vi "Image UDP Broadcast Main Page.vi"(8 "error in (no error)":errorcluster, 11 "Node Ptr":T4 format="%.0x") -> (0 "error out":errorcluster)   [LabVIEW 2012, in "Image UDP Broadcast Custom Device.lvlib"]
uses:
  Shared/Image UDP Broadcast Custom Device.lvlib
  <vilib>/NI Veristand/Custom Device API/Custom Device Item Ref.ctl
  Ctls/Acquisition States.ctl
  Ctls/Acquisition Data.ctl
  <vilib>/userdefined/High Color/IMAQdx.ctl
  <vilib>/vision/Image Controls.llb/IMAQ Image.ctl
  Shared/Image UDP Broadcast Global Variable.vi
  <vilib>/NI Veristand/Custom Device API/Custom Device API.lvlib
  <vilib>/vision/driver/NI_Vision_Acquisition_Software.lvlib
panel:
  out "Valid Bytes per Packet":bool
  in  "Remote IP Address":string
  out "Camera State":T1
  in  "Image Type":T2 items=["Grayscale (U8)", "Grayscale (I16)", "Grayscale (SGL)", "Complex (CSG)", "RGB (U32)", "HSL (U32)", "RGB (U64)", "Grayscale (U16)"]
  in  "Quality":i32 min=0 max=1000 step=5
  out "% Bytes per Packet":dbl
  in  "UDP Port":u16
  in  "Discover IMAQdx":bool
  in  "NI-IMAQdx Devices":i32(listbox)
  in  "Camera Interface":string="cam0"
  in  "Grab":bool
  out "Image":T3(plugin-control)
  in  "Header":cluster{"Section Name":string}={"Section Name"="Custom Device Item Settings"}
  in  "Name":string
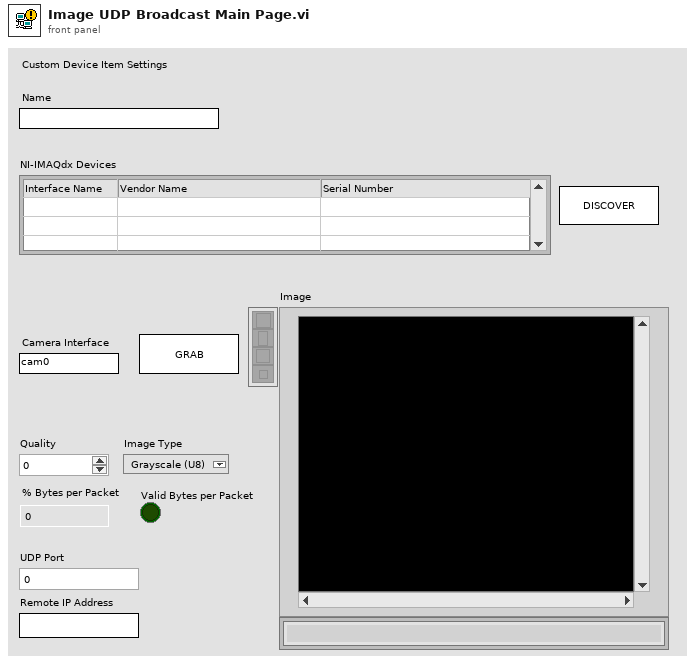
[diagram p1: front panel]
types:
  T1 = typedef "Image UDP Broadcast Custom Device.lvlib/Acquisition States.ctl" = enum8{"Idle", "Init & Config", "Acq", "Stop"}
  T2 = typedef "Image Type" = u32
  T3 = typedef "IMAQ Image.ctl" = refnum<image>
  T4 = typedef "Custom Device API.lvlib/Custom Device Item Ref.ctl" = u64
  T5 = typedef "Image UDP Broadcast Custom Device.lvlib/Acquisition Data.ctl" = cluster{"State":T1, "IMAQdx Session":T6, "Image":T3, "% Bytes per Packet":dbl}
  T6 = typedef "IMAQdx.ctl" = refnum<k21>
  T7 = typedef "Custom Device API.lvlib/Custom Device Item Info.ctl" = cluster{"Name":string, "Is Channel":bool, "GUID":string, "Is Waveform":bool}
  T8 = typedef "Custom Device API.lvlib/Custom Device Commands.ctl" = enum16{"Default", "Item renamed", "Shutdown", "Dynamic button pressed"}
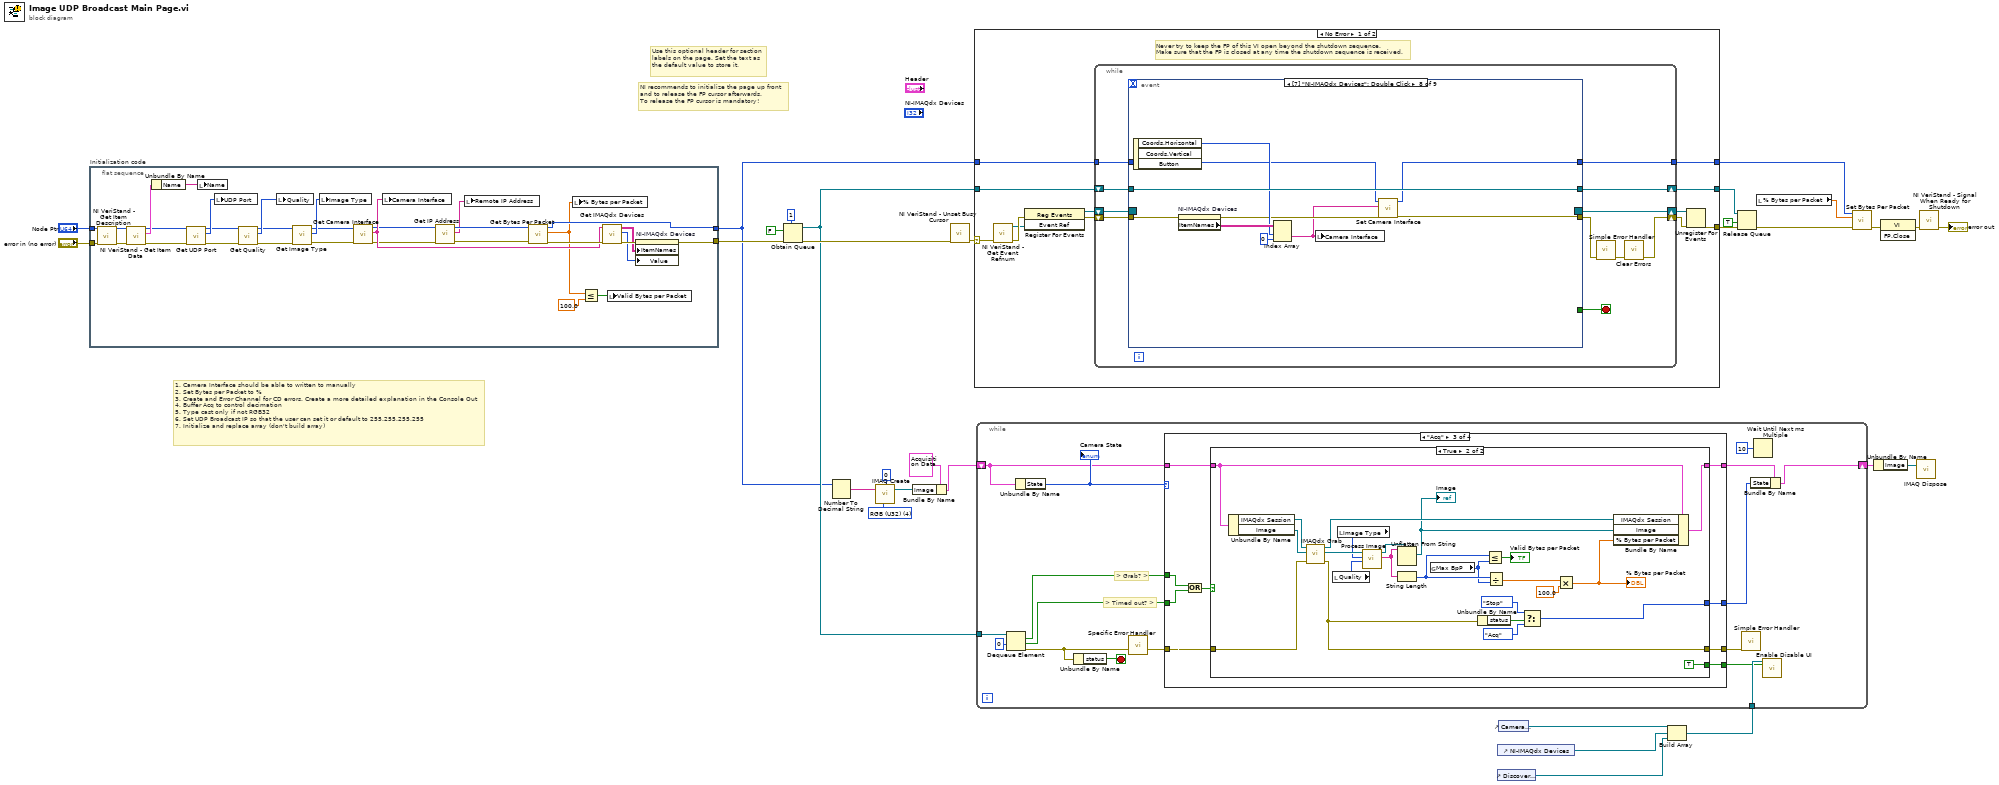
[diagram p0: block diagram]
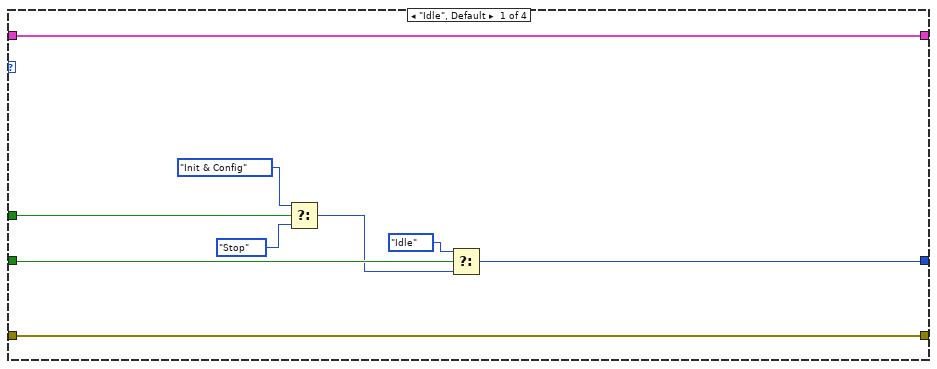
[diagram p2: hidden frame]
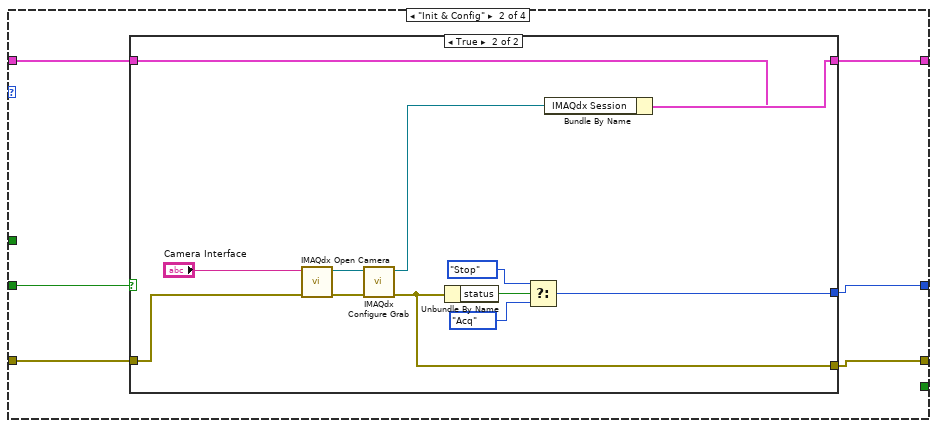
[diagram p3: hidden frame]
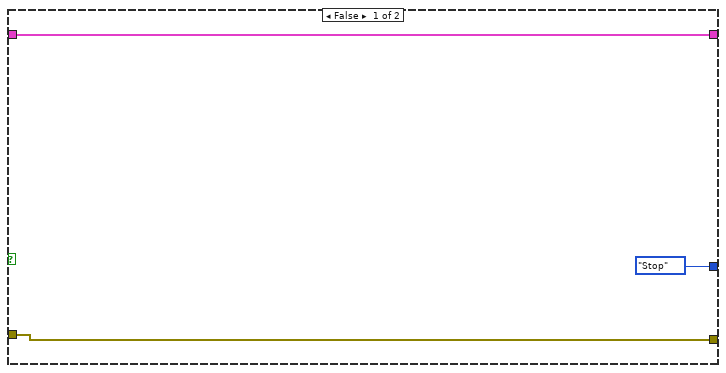
[diagram p4: hidden frame]
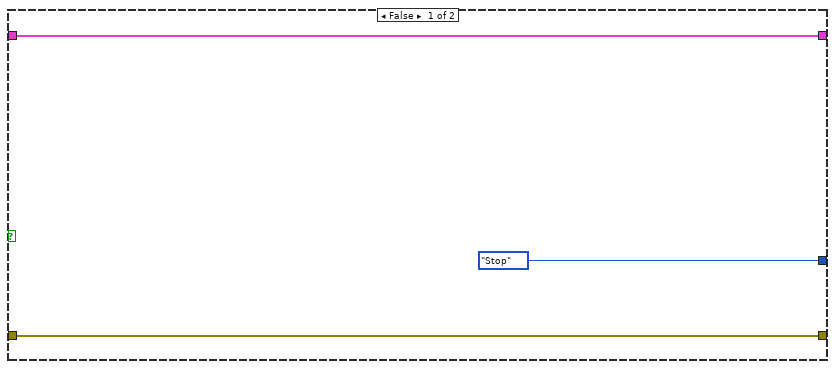
[diagram p5: hidden frame]
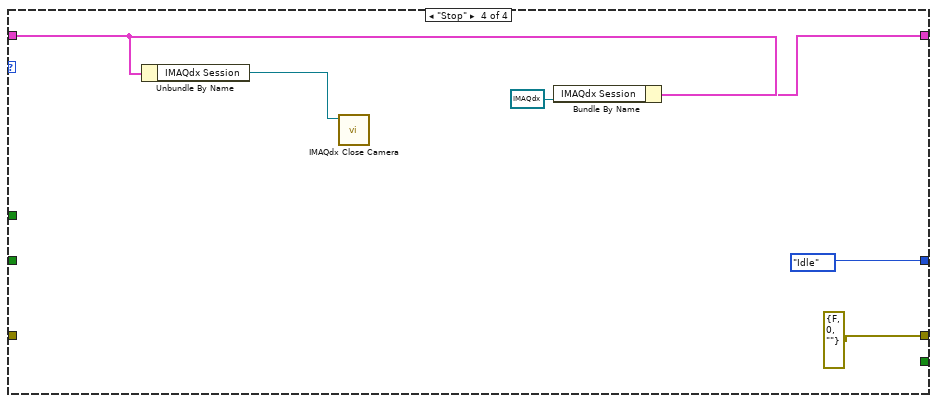
[diagram p6: hidden frame]
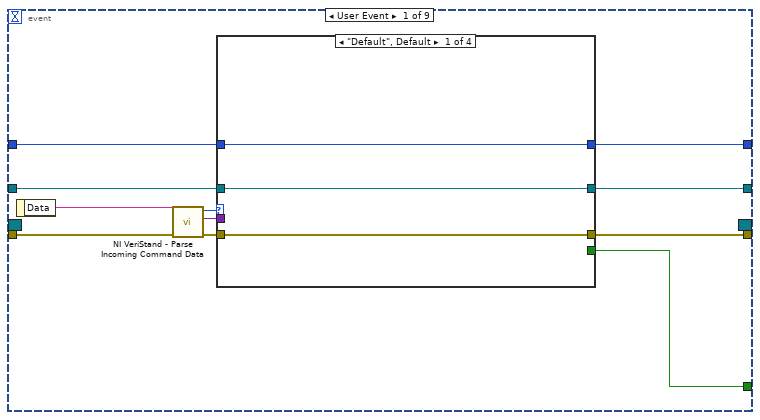
[diagram p7: hidden frame]
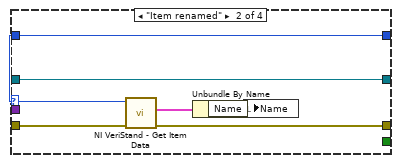
[diagram p8: hidden frame]
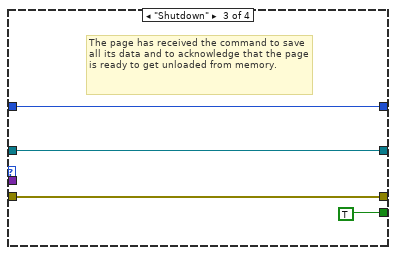
[diagram p9: hidden frame]
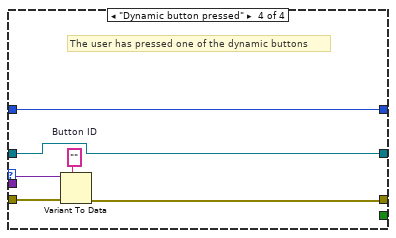
[diagram p10: hidden frame]
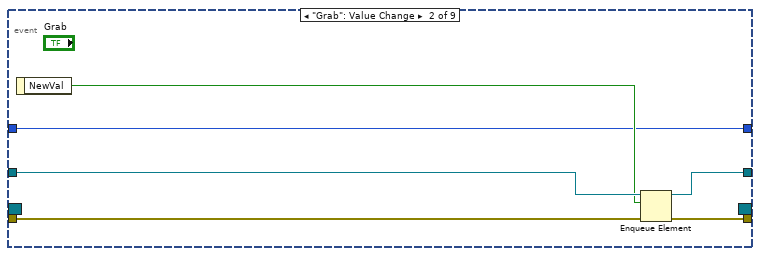
[diagram p11: hidden frame]
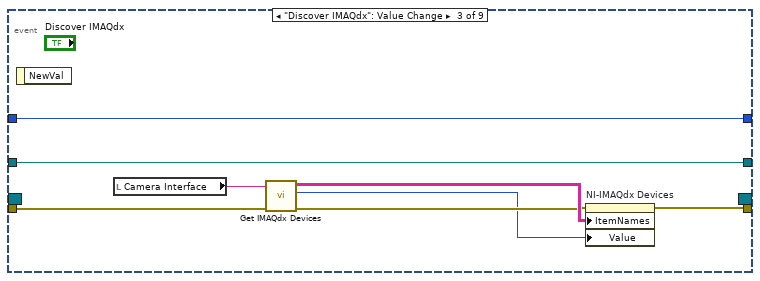
[diagram p12: hidden frame]
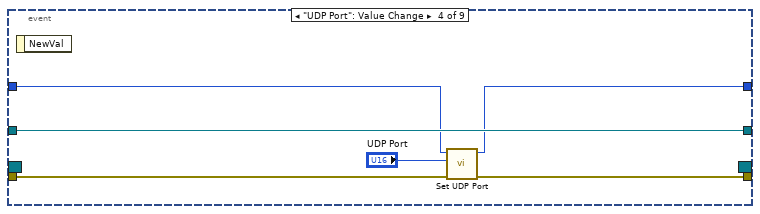
[diagram p13: hidden frame]
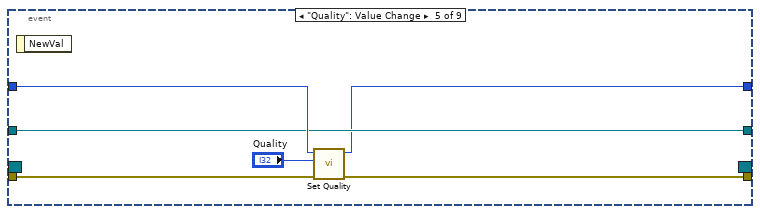
[diagram p14: hidden frame]
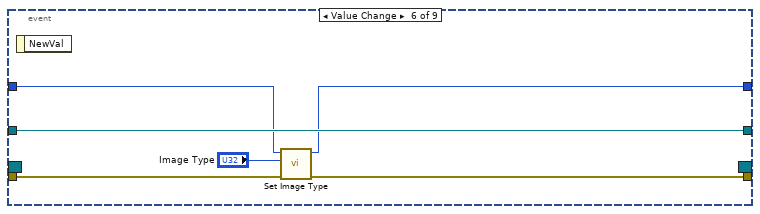
[diagram p15: hidden frame]
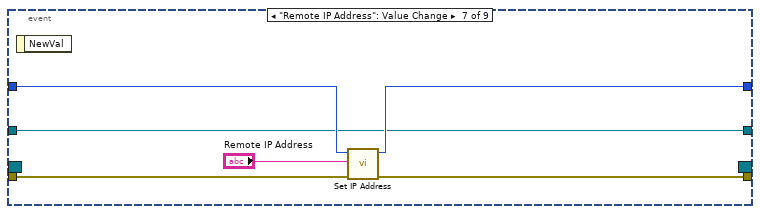
[diagram p16: hidden frame]
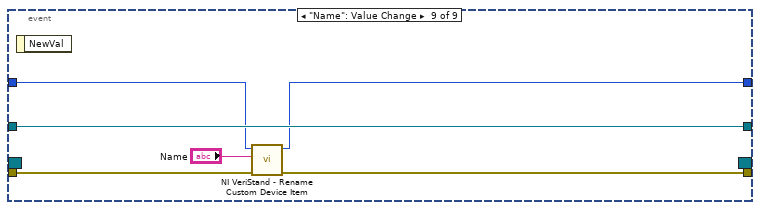
[diagram p17: hidden frame]
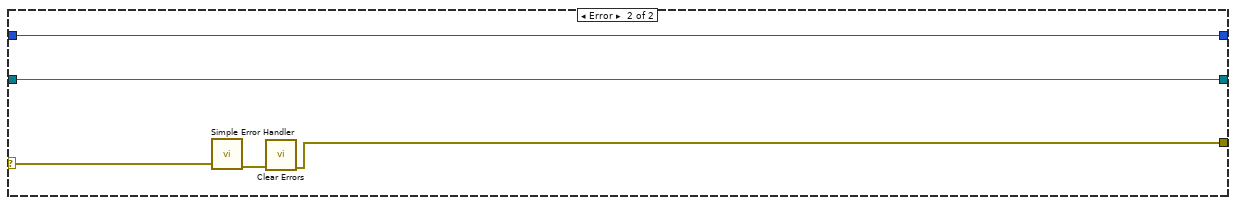
[diagram p18: hidden frame]
diagram:
  w10 = T2 4 items=["Grayscale (U8)", "Grayscale (I16)", "Grayscale (SGL)", "Complex (CSG)", "RGB (U32)", "HSL (U32)", "RGB (U64)", "Grayscale (U16)"] ("Image Type")
  # "1. Camera Interface should be able to written to manually\n2. Set Bytes per Packet to % \n3. Create and Error Channel for CD errors. Create a more detailed explanation in the Console Out\n4. Buffer Acq to control decimation\n5. Type cast only if not RGB32\n6. Set UDP Broadcast IP so that the user can set it or default to 255.255.255.255\n7. Initialize and replace array (don't build array)"
  # "Use this optional header for section labels on the page. Set the text as the default value to store it."
  # "NI recommends to initialize the page up front\nand to release the FP cursor afterwards.\nTo release the FP cursor is mandatory!"
  n1 = flat-sequence "Initialization code" {
    tunnel: "error in (no error)" -> [w60]
    tunnel: "Node Ptr" -> [w59]
    tunnel: [w33] -> w23
    tunnel: [w44] -> w16
    frame #0 {
      n2 = call <vilib>:"NI VeriStand - Get Item Description.vi"("error in (no error)"=w60, "Item Ref in"=w59) -> ("error out"=w58:errorcluster, "Item Ref out"=w61:T4)  [unwired: 8 out]
      n3 = call <vilib>:"NI VeriStand - Get Item Data.vi"("error in (no error)"=w58, "Item Ref in"=w61) -> ("error out"=w54:errorcluster, "Item Info"=w57:T7, "Item Ref out"=w55:T4)  [unwired: 7 out]
      n4 = Unbundle By Name(w57) -> ("Name"=w56:string)
      n5 = call "Get UDP Port.vi"("error in (no error)"=w54, "Dev Ref in"=w55) -> ("error out"=w52:errorcluster, "Value"=w53:u16, "Dev Ref out"=w51:T4)  [unwired: 7 in]
      n6 = local write "Name"(w56) -> ()
      n7 = local write "UDP Port"(w53) -> ()
      n8 = call "Get Quality.vi"("error in (no error)"=w52, "Dev Ref in"=w51) -> ("error out"=w49:errorcluster, "Value"=w50:i32, "Dev Ref out"=w48:T4)  [unwired: 7 in]
      n9 = local write "Quality"(w50) -> ()
      n10 = call "Get Image Type.vi"("error in (no error)"=w49, "Dev Ref in"=w48) -> ("error out"=w45:errorcluster, "Value"=w47:T2, "Dev Ref out"=w46:T4)  [unwired: 7 in]
      n11 = local write "Image Type"(w47) -> ()
      n12 = call "Get Camera Interface.vi"("error in (no error)"=w45, "Dev Ref in"=w46) -> ("error out"=w38:errorcluster, "Value"=w39:string, "Dev Ref out"=w37:T4)  [unwired: 7 in]
      n13 = local write "Camera Interface"(w39) -> ()
      n14 = call "Get IP Address.vi"("error in (no error)"=w38, "Dev Ref in"=w37) -> ("error out"=w35:errorcluster, "Value"=w34:string, "Dev Ref out"=w36:T4)  [unwired: 7 in]
      n15 = local write "Remote IP Address"(w34) -> ()
      n16 = call "Get Bytes Per Packet.vi"("error in (no error)"=w35, "Dev Ref in"=w36) -> ("error out"=w42:errorcluster, "Value"=w32:dbl, "Dev Ref out"=w44:T4)  [unwired: 7 in]
      n17 = local write "% Bytes per Packet"(w32) -> ()
      n18 = Less Or Equal?(x=w32, y=100.0) -> (x <= y?=w30:bool)
      n19 = call "Get IMAQdx Devices.vi"("error in (no error)"=w42, "Chosen Interface"=w39) -> ("error out"=w43:errorcluster, "Row of Chosen Interface"=w40:i32, "IMAQdx Devices"=w41:string[][])  [unwired: 6 in, 1 out]
      n20 = local write "Valid Bytes per Packet"(w30) -> ()
      n21 = property on="NI-IMAQdx Devices" class="MCListbox (strict)"(error in=w43, "ItemNames"=w41, "Value"=w40) -> (error out=w33:errorcluster)  [unwired: 1 in, 1 out]
    }
  }
  n22 = Obtain Queue(max queue size (-1, unlimited)=1, element data type=FALSE ("Grab"), error in (no error)=w23) -> (queue out=w17:refnum<queue>, error out=w18:errorcluster)  [unwired: 2 in, 1 out]
  n23 = Number To Decimal String(number=w16) -> (decimal integer string=w8:string)  [unwired: 1 in]
  n24 = call "IMAQ Create"("Border Size"=0, "Image Name"=w8, "Image Type"=w10) -> ("New Image"=w7:T3)  [unwired: 2 in, 1 out]
  n25 = Bundle By Name(cluster=T5 {"State"=enum."Idle", "IMAQdx Session"="", "Image"=refnum, "% Bytes per Packet"=0.0}, "Image"=w7) -> (w11:T5)
  n26 = call <vilib>:"NI VeriStand - Unset Busy Cursor.vi"("error in (no error)"=w18) -> ("error out"=w26:errorcluster)  [unwired: 10 out]
  n27 = case shown="No Error" w26 {
    selector: w26 -> [w65 w173]
    tunnel: [w70 w171] -> w21
    tunnel: w16 -> [w66 w169]
    tunnel: w17 -> [w64 w170]
    tunnel: [w63 w170] -> w20
    tunnel: [w62 w169] -> w4
    frame No Error {
      # "Never try to keep the FP of this VI open beyond the shutdown sequence.\nMake sure that the FP is closed at any time the shutdown sequence is received."
      n28 = call <vilib>:"NI VeriStand - Get Event Refnum.vi"("error in (no error)"=w65) -> ("error out"=w73:errorcluster, "Event Ref"=w69:refnum<user-event>)  [unwired: 9 out]
      n29 = register-events(error in=w73, w69) -> (reference out=w67:refnum<event-registration>, error out=w68:errorcluster)  [unwired: 1 in]
      n30 = while {
        tunnel: w66 -> [w80]
        shift-right: [w77] -> w71
        shift-left: w68 -> [w83]
        shift-right: [w84] -> w72
        shift-left: w67 -> [w82]
        shift-right: [w75] -> w63
        shift-left: w64 -> [w76]
        tunnel: [w74] -> w62
        stop <- w81 stop-if-true
        n31 = event shown="[7] \"NI-IMAQdx Devices\": Double Click" {
          selector: w82 -> [_ _ _ _ _ _ _ _ _]
          dyn-events: [_ _ _ _ _ _ _ _ _] -> w84
          timeout: _ -> [_ _ _ _ _ _ _ _ _]
          tunnel: w83 -> [w95 w115 w127 w133 w140 w146 w152 w162 w168]
          tunnel: [w91 _ _ _ _ _ _ _ _] -> w81
          tunnel: [w90 w118 w124 w132 w139 w145 w149 w156 w167] -> w79
          tunnel: w80 -> [w89 w116 w123 w131 w138 w143 w151 w154 w164]
          tunnel: w76 -> [w86 w120 w128 w134 w136 w144 w148 w159 w165]
          tunnel: [w85 w119 w128 w134 w136 w144 w148 w159 w165] -> w75
          tunnel: [w87 w116 w123 w129 w135 w141 w150 w153 w163] -> w74
          event User Event {
            n32 = event-data() -> ("Data"=w94:string)  [unwired: 1 out]
            n33 = call <vilib>:"NI VeriStand - Parse Incoming Command Data.vi"("error in (no error)"=w95, "Incoming data"=w94) -> ("error out"=w93:errorcluster, "Outgoing data"=w88:variant, "Action"=w92:T8)  [unwired: 7 out]
            n34 = case shown="\"Default\", Default" w92 {
              tunnel: w93 -> [w98 w104 w105 w114]
              tunnel: [_ _ TRUE _] -> w91
              tunnel: [w98 w102 w105 w111] -> w90
              tunnel: w89 -> [w97 w100 w107 w110]
              tunnel: w88 -> [_ _ _ w113]
              tunnel: [w97 w100 w107 w110] -> w87
              tunnel: w86 -> [w96 w99 w106 w109]
              tunnel: [w96 w99 w106 w109] -> w85
              frame "Default", Default {
              }
              frame "Item renamed" {
                n35 = call <vilib>:"NI VeriStand - Get Item Data.vi"("error in (no error)"=w104, "Item Ref in"=w100) -> ("error out"=w102:errorcluster, "Item Info"=w103:T7)  [unwired: 8 out]
                n36 = Unbundle By Name(w103) -> ("Name"=w101:string)
                n37 = local write "Name"(w101) -> ()
              }
              frame "Shutdown" {
                # "The page has received the command to save all its data and to acknowledge that the page is ready to get unloaded from memory."
              }
              frame "Dynamic button pressed" {
                w112 = ""  # Button ID
                # "The user has pressed one of the dynamic buttons"
                n38 = Variant To Data(error in=w114, type=w112, Variant=w113) -> (error out=w111:errorcluster)  [unwired: 1 out]
              }
            }
          }
          event "Grab": Value Change {
            n39 = event-data() -> ("NewVal"=w117:bool)  [unwired: 1 out]
            n40 = Enqueue Element(queue=w120, element=w117, error in (no error)=w115) -> (queue out=w119:refnum<queue>, error out=w118:errorcluster)  [unwired: 1 in, 1 out]
          }
          event "Discover IMAQdx": Value Change {
            n41 = event-data() -> ()  [unwired: 2 out]
            n42 = local read "Camera Interface"() -> (w121:string)
            n43 = call "Get IMAQdx Devices.vi"("error in (no error)"=w127, "Chosen Interface"=w121) -> ("error out"=w125:errorcluster, "Row of Chosen Interface"=w122:i32, "IMAQdx Devices"=w126:string[][])  [unwired: 6 in, 1 out]
            n44 = property on="NI-IMAQdx Devices" class="MCListbox (strict)"(error in=w125, "ItemNames"=w126, "Value"=w122) -> (error out=w124:errorcluster)  [unwired: 1 in, 1 out]
          }
          event "UDP Port": Value Change {
            n45 = event-data() -> ()  [unwired: 2 out]
            n46 = call "Set UDP Port.vi"("error in (no error)"=w133, "Value"="UDP Port", "Dev Ref in"=w131) -> ("error out"=w132:errorcluster, "Dev Ref out"=w129:T4)  [unwired: 7 in]
          }
          event "Quality": Value Change {
            n47 = event-data() -> ()  [unwired: 2 out]
            n48 = call "Set Quality.vi"("error in (no error)"=w140, "Value"="Quality", "Dev Ref in"=w138) -> ("error out"=w139:errorcluster, "Dev Ref out"=w135:T4)  [unwired: 7 in]
          }
          event Value Change {
            n49 = event-data() -> ()  [unwired: 2 out]
            n50 = call "Set Image Type.vi"("error in (no error)"=w146, "Value"="Image Type", "Dev Ref in"=w143) -> ("error out"=w145:errorcluster, "Dev Ref out"=w141:T4)  [unwired: 7 in]
          }
          event "Remote IP Address": Value Change {
            n51 = event-data() -> ()  [unwired: 2 out]
            n52 = call "Set IP Address.vi"("error in (no error)"=w152, "Value"="Remote IP Address", "Dev Ref in"=w151) -> ("error out"=w149:errorcluster, "Dev Ref out"=w150:T4)  [unwired: 7 in]
          }
          event "NI-IMAQdx Devices": Double Click {
            n53 = event-data() -> ("Coords.Horizontal"=w158:i32)  [unwired: 3 out]
            n54 = property on="NI-IMAQdx Devices" class="MCListbox (strict)"(error in=w162) -> (error out=w157:errorcluster, "ItemNames"=w161:string[][])  [unwired: 1 in, 1 out]
            n55 = Index Array(array=w161, index (row)=w158, index (col)=0 ("disabled index (col)")) -> (element=w155:string)
            n56 = local write "Camera Interface"(w155) -> ()
            n57 = call "Set Camera Interface.vi"("error in (no error)"=w157, "Value"=w155, "Dev Ref in"=w154) -> ("error out"=w156:errorcluster, "Dev Ref out"=w153:T4)  [unwired: 7 in]
          }
          event "Name": Value Change {
            n58 = event-data() -> ()  [unwired: 2 out]
            n59 = call <vilib>:"NI VeriStand - Rename Custom Device Item.vi"("error in (no error)"=w168, "New Name"="Name", "Item Ref in"=w164) -> ("error out"=w167:errorcluster, "Item Ref out"=w163:T4)  [unwired: 1 in, 6 out]
          }
        }
        n60 = call <vilib>:"Simple Error Handler.vi"("error in (no error)"=w79) -> ("error out"=w78:errorcluster)  [unwired: 1 in, 7 out]
        n61 = call <vilib>:"Clear Errors.vi"("error in (no error)"=w78) -> ("error out"=w77:errorcluster)  [unwired: 6 out]
      }
      n62 = Unregister For Events(event registration refnum=w72, error in=w71) -> (error out=w70:errorcluster)
    }
    frame Error {
      n63 = call <vilib>:"Simple Error Handler.vi"("error in (no error)"=w173) -> ("error out"=w172:errorcluster)  [unwired: 1 in, 7 out]
      n64 = call <vilib>:"Clear Errors.vi"("error in (no error)"=w172) -> ("error out"=w171:errorcluster)  [unwired: 6 out]
    }
  }
  n65 = control-ref of="NI-IMAQdx Devices"() -> (w14:refnum<vi>)
  n66 = control-ref of="Discover IMAQdx"() -> (w13:refnum<vi>)
  n67 = control-ref of="Camera Interface"() -> (w15:refnum<vi>)
  n68 = Build Array(w15, w14, w13) -> (w2:refnum<vi>[])
  n69 = while {
    tunnel: w17 -> [w188]
    shift-right: [w181] -> w6
    shift-left: w11 -> [w178]
    tunnel: w2 -> [w175]
    stop <- w184 stop-if-true
    # "> Grab? >"
    # "> Timed out? >"
    n70 = Dequeue Element(queue=w188, timeout in ms (-1)=0) -> (element=w185:bool, timed out?=w186:bool, error out=w177:errorcluster)  [unwired: 1 in, 1 out]
    n71 = Unbundle By Name(w178) -> ("State"=w179:T1)
    "Camera State" <- w179
    n72 = Unbundle By Name(w177) -> ("status"=w184:bool)
    n73 = call "Specific Error Handler"("Error to Check"=w177) -> ("error out"=w176:errorcluster)  [unwired: 11 in, 3 out]
    n74 = case shown="\"Acq\"" w179 {
      tunnel: w186 -> [w198 w203 w227 _]
      tunnel: w176 -> [w191 w204 w228 _]
      tunnel: w185 -> [w196 _ w225 _]
      tunnel: w178 -> [w190 w202 w223 w259]
      tunnel: [w190 w201 w222 w258] -> w183
      tunnel: [w192 w200 w224 Acquisition_States."Idle"] -> w182
      tunnel: [w191 w199 w221 errorcluster {"status"=FALSE, "code"=0, "source"=""} ("error out")] -> w180
      tunnel: [_ _ w220 _] -> w174
      frame "Idle", Default {
        n75 = Select(t=Acquisition_States."Init & Config", s=w196, f=Acquisition_States."Stop") -> (s? t:f=w193:T1)
        n76 = Select(t=Acquisition_States."Idle", s=w198, f=w193) -> (s? t:f=w192:T1)
      }
      frame "Init & Config" {
        n77 = case shown="True" w203 {
          tunnel: w204 -> [w206 w217]
          tunnel: [Acquisition_States."Stop" w216] -> w200
          tunnel: w202 -> [w205 w208]
          tunnel: [w205 w215] -> w201
          tunnel: [w206 w212] -> w199
          frame False {
          }
          frame True {
            n78 = call <vilib>:"IMAQdx Open Camera.vi"("error in"=w217, "Session In"="Camera Interface") -> ("error out"=w214:errorcluster, "Session Out"=w213:T6)  [unwired: 8 in]
            n79 = call <vilib>:"IMAQdx Configure Grab.vi"("error in"=w214, "Session In"=w213) -> ("error out"=w212:errorcluster, "Session Out"=w210:T6)  [unwired: 8 in]
            n80 = Unbundle By Name(w212) -> ("status"=w211:bool)
            n81 = Select(t=Acquisition_States."Stop", s=w211, f=Acquisition_States."Acq") -> (s? t:f=w216:T1)
            n82 = Bundle By Name(cluster=w208, "IMAQdx Session"=w210) -> (w215:T5)
          }
        }
      }
      frame "Acq" {
        n83 = Or(x=w225, y=w227) -> (x .or. y?=w226:bool)
        n84 = case shown="True" w226 {
          tunnel: w228 -> [w230 w253]
          tunnel: [Acquisition_States."Stop" w247] -> w224
          tunnel: w223 -> [w229 w252]
          tunnel: [w229 w251] -> w222
          tunnel: [w230 w246] -> w221
          tunnel: [_ TRUE ("Disable?")] -> w220
          frame False {
          }
          frame True {
            n85 = Unbundle By Name(w252) -> ("IMAQdx Session"=w255:T6, "Image"=w254:T3)
            n86 = call <vilib>:"IMAQdx Grab.vi"("error in"=w253, "Image In"=w254, "Session In"=w255) -> ("error out"=w246:errorcluster, "Image Out"=w243:T3, "Session Out"=w250:T6)  [unwired: 5 in, 1 out]
            n87 = local read "Quality"() -> (w239:i32)
            n88 = local read "Image Type"() -> (w240:T2)
            n89 = call "Process Image.vi"("Quality"=w239, "Image Type"=w240, "Image in"=w243) -> ("Data String"=w244:string, "Image out"=w242:T3)  [unwired: 6 in, 1 out]
            n90 = Unflatten From String(type=w242, binary string=w244) -> (value=w241:T3)  [unwired: 3 in, 2 out]
            "Image" <- w241
            n91 = String Length(string=w244) -> (length=w234:i32)
            n92 = global read "Image UDP Broadcast Global Variable.vi" "Max BpP"() -> (w233:i32)
            n93 = Unbundle By Name(w246) -> ("status"=w245:bool)
            n94 = Less Or Equal?(x=w234, y=w233) -> (x <= y?=→"Valid Bytes per Packet":bool)
            n95 = Divide(x=w234, y=w233) -> (x/y=w236:dbl)
            n96 = Select(t=Acquisition_States."Stop", s=w245, f=Acquisition_States."Acq") -> (s? t:f=w247:T1)
            n97 = Multiply(x=w236, y=100.0) -> (x*y=w235:dbl)
            "% Bytes per Packet" <- w235
            n98 = Bundle By Name(cluster=w252, "IMAQdx Session"=w250, "Image"=w241, "% Bytes per Packet"=w235) -> (w251:T5)
          }
        }
      }
      frame "Stop" {
        n99 = Unbundle By Name(w259) -> ("IMAQdx Session"=w260:T6)
        n100 = call <vilib>:"IMAQdx Close Camera.vi"("Session In"=w260) -> ()  [unwired: 10 in, 1 out]
        n101 = Bundle By Name(cluster=w259, "IMAQdx Session"=T6 refnum) -> (w258:T5)
      }
    }
    n102 = call <vilib>:"Simple Error Handler.vi"("error in (no error)"=w180) -> ()  [unwired: 4 in, 5 out]
    n103 = Bundle By Name(cluster=w183, "State"=w182) -> (w181:T5)
    n104 = Wait Until Next ms Multiple(millisecond multiple=u32 10) -> ()  [unwired: 1 out]
    n105 = call "Enable Disable UI.vi"("Disable?"=w174, "Reference Array in"=w175) -> ()  [unwired: 8 in, 2 out]
  }
  n106 = Release Queue(queue=w20, force destroy? (F)=TRUE, error in (no error)=w21) -> (error out=w3:errorcluster)  [unwired: 2 out]
  n107 = local read "% Bytes per Packet"() -> (w1:dbl)
  n108 = call "Set Bytes Per Packet.vi"("Value"=w1, "Dev Ref in"=w4) -> ()  [unwired: 8 in, 2 out]
  n109 = Unbundle By Name(w6) -> ("Image"=w5:T3)
  n110 = invoke class="VI" method="FP.Close"(error in=w3) -> (error out=w29:errorcluster)  [unwired: 2 in, 2 out]
  n111 = call "IMAQ Dispose"("Image"=w5) -> ()  [unwired: 5 in, 1 out]
  n112 = call <vilib>:"NI VeriStand - Signal When Ready for Shutdown.vi"("error in (no error)"=w29) -> ("error out"=→"error out":errorcluster)  [unwired: 10 out]
